vi "Any_Char_Replace.vi"(1 "Replace with":string, 2 "Characters to replace":string, 3 "String in":string) -> (0 "String out":string)   [LabVIEW 2012]
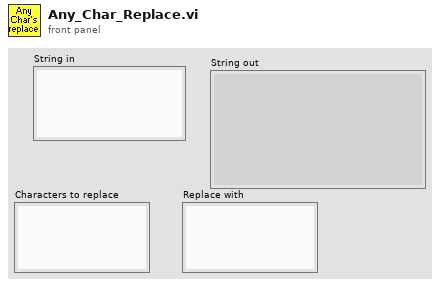
[diagram p1: front panel]
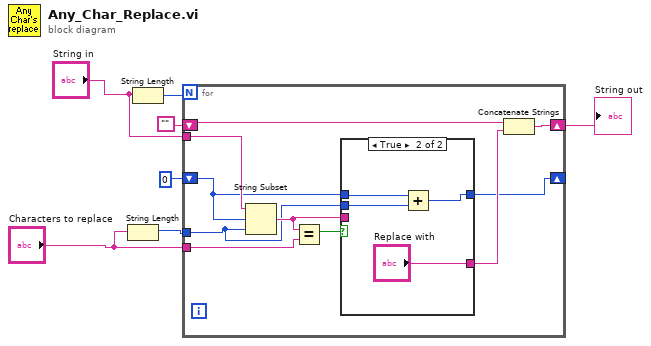
[diagram p0: block diagram]
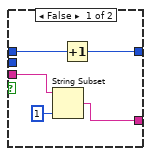
[diagram p2: hidden frame]
diagram:
  n1 = String Length(string="Characters to replace") -> (length=w2:i32)
  n2 = String Length(string="String in") -> (length=w4:i32)
  n3 = for {
    N: w4 -> [_]
    tunnel: "String in" -> [w17]
    tunnel: "Characters to replace" -> [w16]
    shift-right: [w14] -> w7
    shift-left: "" -> [w15]
    tunnel: w2 -> [w8]
    shift-right: [w9] -> _
    shift-left: 0 -> [w10]
    n4 = String Subset(string=w17, offset (0)=w10, length (rest)=w8) -> (substring=w11:string)
    n5 = Equal?(x=w11, y=w16) -> (x = y?=w13:bool)
    n6 = case shown="True" w13 {
      tunnel: [w20 "Replace with"] -> w12
      tunnel: w11 -> [w21 _]
      tunnel: w10 -> [w19 w25]
      tunnel: [w18 w24] -> w9
      tunnel: w8 -> [_ w23]
      frame False {
        n7 = String Subset(string=w21, length (rest)=1 ("length (rest)")) -> (substring=w20:string)  [unwired: 1 in]
        n8 = Increment(x=w19) -> (x+1=w18:i32)
      }
      frame True {
        n9 = Add(x=w25, y=w23) -> (x+y=w24:i32)
      }
    }
    n10 = Concatenate Strings(w15, w12) -> (w14:string)
  }
  "String out" <- w7
